vi "FTW-Endpoint-Pipe-Flush.vi"(0 "FTW Endpoint":refnum<class "FTW-Endpoint.lvclass">, 11 "error in":errorcluster) -> (4 "FTW Endpoint out":refnum<class "FTW-Endpoint.lvclass">, 15 "error out":errorcluster)   [LabVIEW 2015, in "FTW-Endpoint.lvclass"]
uses:
  FTW-Endpoint.lvclass
  FTW-Endpoint.lvclass/FTW-Endpoint.ctl
panel:
  # "Inputs"
  # "Outputs"
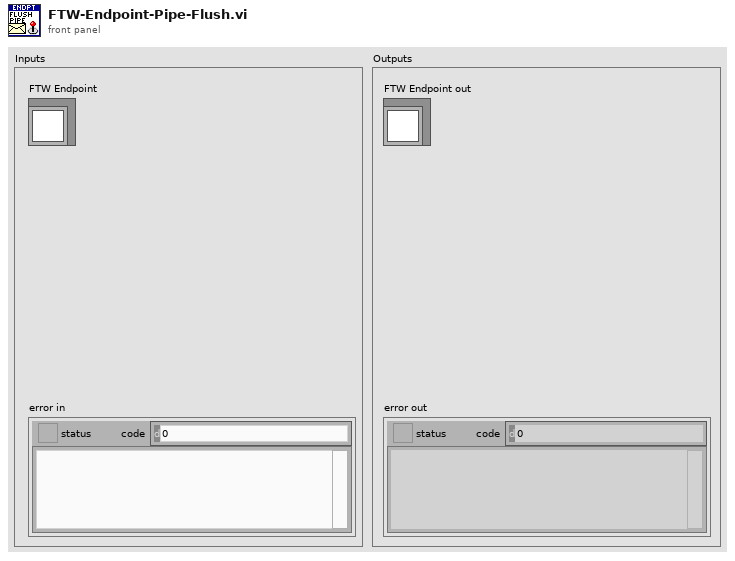
[diagram p1: front panel]
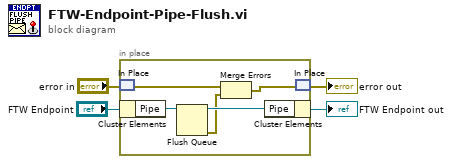
[diagram p0: block diagram]
diagram:
  n1 = in-place {
    n2 = in-place-match #1("error in") -> (w6:errorcluster)
    n3 = in-place-cluster #2("FTW Endpoint") -> ("Pipe"=w7:refnum<queue>)
    n4 = Flush Queue(queue=w7) -> (queue out=w9:refnum<queue>, error out=w8:errorcluster)  [unwired: 1 in, 1 out]
    n5 = Merge Errors(w6, w8) -> (w5:errorcluster)
    n6 = in-place-cluster #2("Pipe"=w9) -> (→"FTW Endpoint out":refnum<class "FTW-Endpoint.lvclass">)
    n7 = in-place-match #1(w5) -> (→"error out":errorcluster)
  }
